vi "ToggleLights.vi"(0 "reference in":refnum<class "LightingSystem.lvclass">, 2 "RoomName":string, 5 "Error In":errorcluster) -> (14 "reference out":refnum<class "LightingSystem.lvclass">, 19 "Error Out":errorcluster)   [LabVIEW 2024, in "LightingSystem.lvclass"]
uses:
  LightingSystem.lvclass
  LightingSystem.lvclass/LightingSystem.ctl
  House/Room_class/Room.lvclass
  Devices/Light_class/Light.lvclass
panel:
  # "Connector Pane"
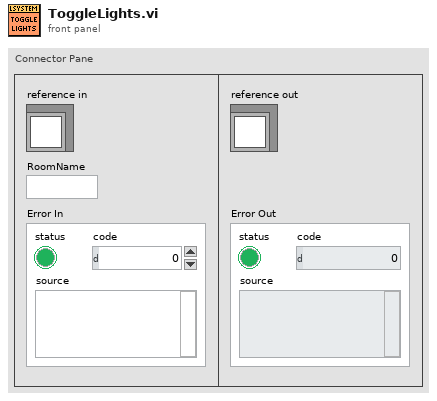
[diagram p1: front panel]
types:
  T1 = typedef "LightingSystem.lvclass/ObjectAttributes.ctl" = cluster{"Rooms":T2}
  T2 = typedef "Rooms Map.ctl" = map{string, refnum<class "Room.lvclass">}
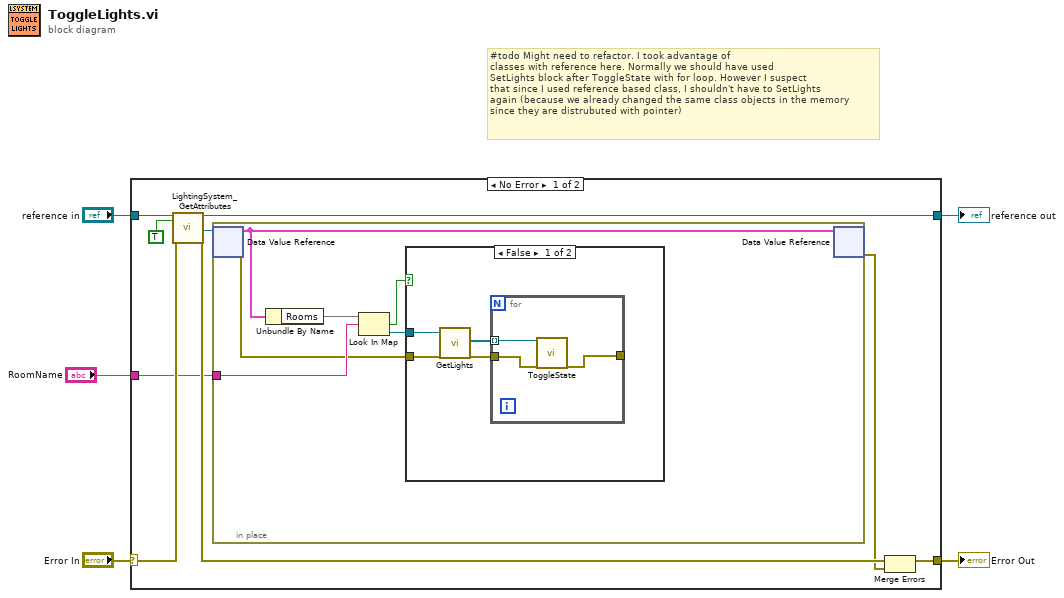
[diagram p0: block diagram]
diagram:
  # "#todo Might need to refactor. I took advantage of\nclasses with reference here. Normally we should have used\nSetLights block after ToggleState with for loop. However I suspect\nthat since I used reference based class, I shouldn't have to SetLights\nagain (because we already changed the same class objects in the memory\nsince they are distrubuted with pointer)"
  n1 = case shown="No Error" "Error In" {
    selector: "Error In" -> [w13 w29]
    tunnel: [w11 w29] -> w4
    tunnel: [w12 w28] -> w2
    tunnel: "reference in" -> [w14 w28]
    tunnel: "RoomName" -> [w6 _]
    frame No Error {
      n2 = call "LightingSystem_GetAttributes.vi"("reference in"=w14, "OnlyGetDvrReference(False)"=TRUE, "Error In"=w13) -> ("reference out"=w12:refnum<class "LightingSystem.lvclass">, "DataRef"=w10:refnum<data-value>, "Error Out"=w8:errorcluster)  [unwired: 13 in, 1 out]
      n3 = in-place {
        in-place-border: w6 -> [w18]
        n4 = in-place-dvr #1(w10) -> (w20:T1, w15:errorcluster)
        n5 = Unbundle By Name(w20) -> ("Rooms"=w19:T2)
        n6 = Look In Map(map=w19, key=w18) -> (key not found?=w17:bool, value=w16:refnum<class "Room.lvclass">)  [unwired: 1 in]
        n7 = case shown="False" w17 {
          tunnel: w16 -> [w24 _]
          tunnel: w15 -> [w21 _]
          frame False {
            n8 = call-dynamic "GetLights.vi"("reference in"=w24, "Error In"=w21) -> ("Lights"=w23:refnum<class "Light.lvclass">[], "Error Out"=w22:errorcluster)  [unwired: 15 in, 1 out]
            n9 = for {
              tunnel: w23 -> [w27] mode=indexing
              tunnel: w22 -> [w26]
              tunnel: [w25] -> _
              n10 = call "ToggleState.vi"("reference in"=w27, "Error In"=w26) -> ("Error Out"=w25:errorcluster)  [unwired: 16 in, 1 out]
            }
          }
          frame True {
          }
        }
        n11 = in-place-dvr #1(w20) -> (w7:errorcluster)  [unwired: 1 out]
      }
      n12 = Merge Errors(w8, w7) -> (w11:errorcluster)
    }
    frame Error {
    }
  }
  "Error Out" <- w4
  "reference out" <- w2
